vi "Crosspoint.vi"(8 "error in (no error)":errorcluster, 11 "Trace In":refnum<class "Trace.lvclass">) -> (0 "error out":errorcluster)   [LabVIEW 2021, in "Trace.lvclass"]
uses:
  Trace.lvclass
panel:
  in  "Trace 2":refnum<class "Trace.lvclass">
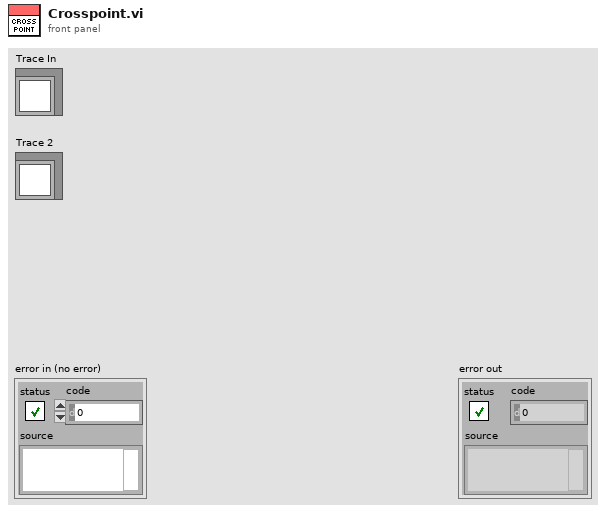
[diagram p1: front panel]
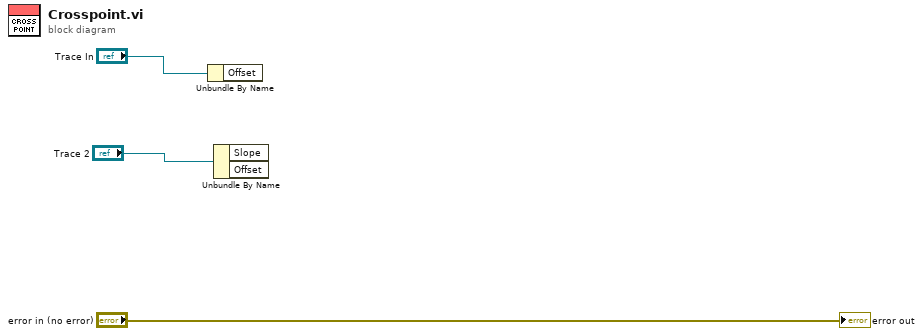
[diagram p0: block diagram]
diagram:
  n1 = Unbundle By Name("Trace In") -> ()  [unwired: 1 out]
  n2 = Unbundle By Name("Trace 2") -> ()  [unwired: 2 out]
  "error out" <- "error in (no error)"
